vi "Set External_Trigger.vi"(7 "Simulation":T1, 8 "error in":errorcluster, 9 "String":string, 10 "Args":string[](array[string]), 11 "Ophir Pulsar in":refnum<class "Ophir Juno.lvclass">) -> (0 "error out":errorcluster, 2 "new commands":string, 3 "Ophir Pulsar out":refnum<class "Ophir Juno.lvclass">)   [LabVIEW 2013, in "Ophir Juno.lvclass"]
uses:
  Ophir Juno.lvclass
  shared/OnOffTypeDef.ctl
  Controls/External_Trigger.ctl
  Ophir Juno.lvclass/Ophir Juno.ctl
  shared/CompressAndUpdate(Poly)/CompressAndUpdate(Enum).vi
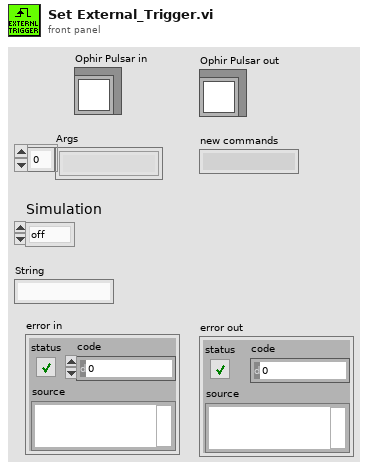
[diagram p1: front panel]
types:
  T1 = typedef "OnOffTypeDef.ctl" = enum16{"off", "on"}
  T2 = typedef "Ophir Juno.lvclass/External_Trigger.ctl" = enum16{"off", "on"}
  T3 = cluster{"Channel0":T2, "Channel1":enum16{"off", "on"}, "Channel2":enum16{"off", "on"}, "Channel3":enum16{"off", "on"}}
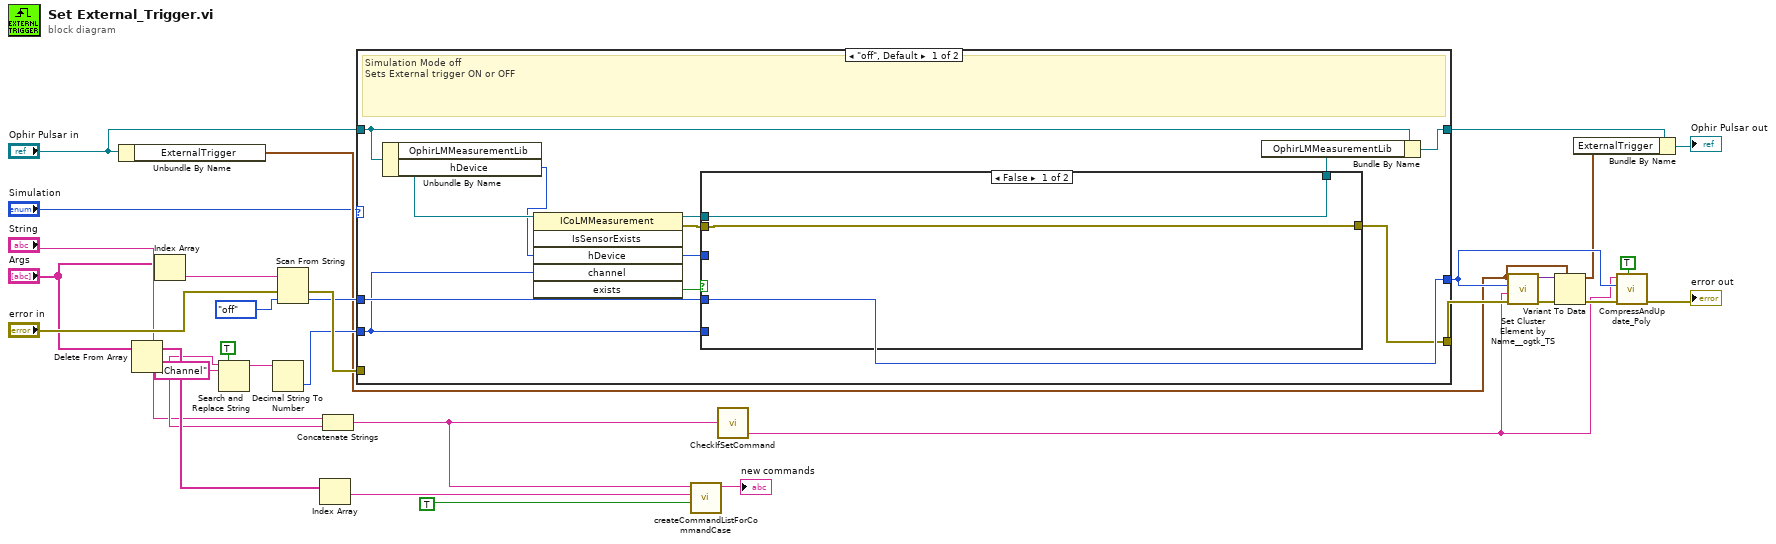
[diagram p0: block diagram]
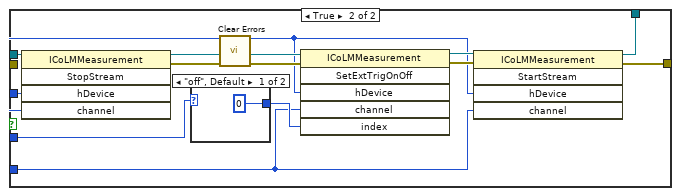
[diagram p2: hidden frame]
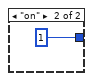
[diagram p3: hidden frame]
diagram:
  n1 = Unbundle By Name("Ophir Pulsar in") -> ("ExternalTrigger"=w12:T3)
  n2 = Delete From Array(array="Args") -> (deleted portion=w10:string, array with subset deleted=w16:string[])  [unwired: 2 in]
  n3 = Index Array(array="Args") -> (element=w22:string)  [unwired: 1 in]
  n4 = Search and Replace String(replace all?=TRUE ("replace all? (F)"), input string=w10, search string=".Channel") -> (result string=w14:string)  [unwired: 5 in, 3 out]
  n5 = Decimal String To Number(string=w14) -> (number=w29:i32)  [unwired: 2 in, 1 out]
  n6 = Scan From String(input string=w22, error in="error in", default 1=External_Trigger."off") -> (error out=w31:errorcluster, output 1=w23:T2)  [unwired: 2 in, 2 out]
  n7 = Index Array(array=w16) -> (element=w17:string)  [unwired: 1 in]
  n8 = Concatenate Strings("String", w10) -> (w15:string)
  n9 = case shown="\"off\", Default" "Simulation" {
    tunnel: w23 -> [w40 w61]
    tunnel: [w40 w61] -> w25
    tunnel: w31 -> [_ w60]
    tunnel: [w39 w60] -> w26
    tunnel: "Ophir Pulsar in" -> [w42 w59]
    tunnel: [w41 w59] -> w19
    tunnel: w29 -> [w34 _]
    frame "off", Default {
      # "Simulation Mode off\nSets External trigger ON or OFF"
      n10 = Unbundle By Name(w42) -> ("OphirLMMeasurementLib"=w37:refnum<k7>, "hDevice"=w35:i32)
      n11 = invoke class="ICoLMMeasurement" method="IsSensorExists"(reference=w37, "hDevice"=w35, "channel"=w34) -> (reference out=w36:refnum<k7>, error out=w32:errorcluster, "exists"=w33:bool)  [unwired: 3 in, 3 out]
      n12 = case shown="False" w33 {
        tunnel: w40 -> [_ w56]
        tunnel: [w43 w50] -> w39
        tunnel: [w44 w49] -> w38
        tunnel: w36 -> [w44 w47]
        tunnel: w35 -> [_ w46]
        tunnel: w34 -> [_ w45]
        tunnel: w32 -> [w43 _]
        frame False {
        }
        frame True {
          n13 = invoke class="ICoLMMeasurement" method="StopStream"(reference=w47, "hDevice"=w46, "channel"=w45) -> (reference out=w53:refnum<k7>, error out=w54:errorcluster)  [unwired: 2 in, 3 out]
          n14 = case shown="\"off\", Default" w56 {
            tunnel: [0 1] -> w55
            frame "off", Default {
            }
            frame "on" {
            }
          }
          n15 = call <vilib>:"Clear Errors.vi"("error in (no error)"=w54) -> ("error out"=w48:errorcluster)  [unwired: 6 in]
          n16 = invoke class="ICoLMMeasurement" method="SetExtTrigOnOff"(reference=w53, error in=w48, "hDevice"=w46, "channel"=w45, "index"=w55) -> (reference out=w52:refnum<k7>, error out=w51:errorcluster)  [unwired: 1 in, 4 out]
          n17 = invoke class="ICoLMMeasurement" method="StartStream"(reference=w52, error in=w51, "hDevice"=w46, "channel"=w45) -> (reference out=w49:refnum<k7>, error out=w50:errorcluster)  [unwired: 1 in, 3 out]
        }
      }
      n18 = Bundle By Name(cluster=w42, "OphirLMMeasurementLib"=w38) -> (w41:refnum<class "Ophir Juno.lvclass">)
    }
    frame "on" {
      # "Simulation Mode on"
    }
  }
  n19 = call "createCommandListForCommandCase.vi"("immediate Check (only once)"=TRUE, "setvalue"=w17, "command"=w15) -> ("new commands"=→"new commands":string)  [unwired: 8 in]
  n20 = call "CheckIfSetCommand.vi"("Command"=w15) -> ("variable"=w9:string)  [unwired: 2 out]
  n21 = call "Set Cluster Element by Name__ogtk_TS.vi"("error in (no error)"=w26, "Element Name (\"\": New Element Data Name)"=w9, "New Element Value"=w25, "Cluster"=w12) -> ("error out"=w27:errorcluster, "VCluster out"=w13:variant)  [unwired: 5 in, 1 out]
  n22 = Variant To Data(error in=w27, type=w12, Variant=w13) -> (data=w11:T3, error out=w28:errorcluster)
  n23 = Bundle By Name(cluster=w19, "ExternalTrigger"=w11) -> (→"Ophir Pulsar out":refnum<class "Ophir Juno.lvclass">)
  n24 = call-poly "CompressAndUpdate_Poly.vi"("force CVT update (false)"=TRUE, "error in"=w28, "enum variant"=w25, "command or variable name"=w9) -> ("error out"=→"error out":errorcluster)  [unwired: 7 in]
